vi "set_volume_leds.vi"(8 "error in (no error)":errorcluster, 9 "Array":dbl[](array[numeric]), 10 "Numeric":i32=10, 11 "Refnum in":refnum<k21>) -> (0 "error out":errorcluster, 2 "Boolean array":bool[](array[boolean]), 3 "Refnum out":refnum<k21>)   [LabVIEW 2022 SP3]
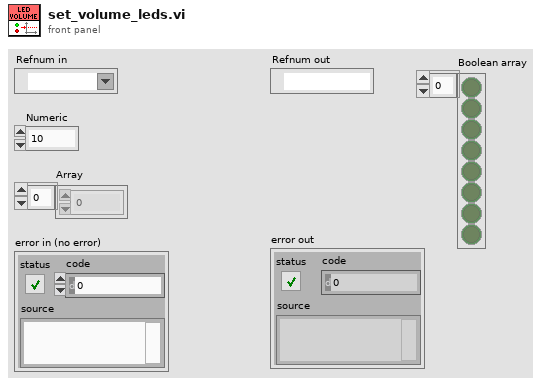
[diagram p1: front panel]
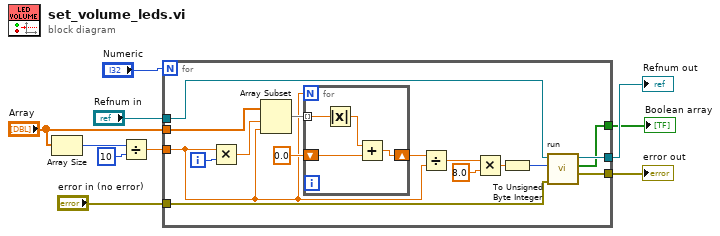
[diagram p0: block diagram]
diagram:
  n1 = Array Size(array="Array") -> (size(s)=w8:i32)
  n2 = Divide(x=w8, y=10) -> (x/y=w6:dbl)
  n3 = for {
    N: "Numeric" -> [_]
    tunnel: "Array" -> [w26]
    tunnel: w6 -> [w13]
    tunnel: "Refnum in" -> [w17]
    tunnel: "error in (no error)" -> [w16]
    tunnel: [w15] -> w3
    tunnel: [w14] -> w2
    tunnel: [w11] -> w1
    i -> [w25]
    n4 = Multiply(x=w13, y=w25) -> (x*y=w24:dbl)
    n5 = Array Subset(array=w26, index=w24, length=w13) -> (w23:dbl[])
    n6 = for {
      N: w13 -> [_]
      tunnel: w23 -> [w28] mode=indexing
      shift-right: [w29] -> w21
      shift-left: 0.0 -> [w30]
      n7 = Absolute Value(x=w28) -> (abs(x)=w27:dbl)
      n8 = Add(x=w27, y=w30) -> (x+y=w29:dbl)
    }
    n9 = Divide(x=w21, y=w13) -> (x/y=w20:dbl)
    n10 = Multiply(x=w20, y=8.0) -> (x*y=w18:dbl)
    n11 = To Unsigned Byte Integer(number=w18) -> (unsigned 8bit integer=w12:u8)
    n12 = call "run.vi"("error in (no error)"=w16, "volume"=w12, "Refnum in"=w17) -> ("error out"=w14:errorcluster, "Array"=w11:bool[], "Refnum out"=w15:refnum<k21>)  [unwired: 6 in]
  }
  "Refnum out" <- w3
  "error out" <- w2
  "Boolean array" <- w1
